vi "AxisSaveConfToFile.vi"(6 "Comunication":T1={"DeviceIDCtrl"=1, "ProtocolCtrl"=enum."Modbus RTU", "COMportCtrl"="", "IPCtrl"=""}, 7 "conf file path":path caption="selected path", 8 "error in (no error)":errorcluster, 9 "AditionalConfigOut":T2 {"UnitsControl" items=["mm", "°"]}, 10 "AxisWriteValuesIn":T3={"AxisTarget"=0.0, "AxisTargetVel"=1.0, "AxisStartReq"=FALSE, "AxisStopReq"=FALSE, "AxisClearReq"=FALSE, "AxisMovetype"=FALSE, "AxisMotorON"=FALSE, "MoveModeControl"=4, "AxisHomingVel"=1.0, "AxisAccDecc"=30.0} {"MoveModeControl" items=["Absolute", "Relative", "Velocity", "Homing"]}, 11 "AxisConfigurationIn":T4={"AxisHomeType"=1, "AxisBacklash"=0.0, "AxisGain"=1.0, "AxisOffset"=0.0, "AxisUnit"=1, "ReqConfRead"=FALSE, "ReqConfWrite"=FALSE, "AxisName"="", "AxisAccDecc"=0.0, "AxisHomeVel"=0.0} {"AxisUnit" items=["mm", "°"]; "AxisHomeType" items=["no homing"=0, "forward limit switch"=1, "backward limit switch"=2, "forward reference"=4, "backward reference"=8]}) -> (0 "error out":errorcluster)   [LabVIEW 2020, in "SMCD14_lib.lvlib"]
uses:
  SMCD14_lib.lvlib
  AxisConfiguration_typedef.ctl
  AxisWriteValues_typedef.ctl
  <vilib>/Utility/config.llb/Write Key (String).vi
  <vilib>/Utility/config.llb/Write Key (U32).vi
  <vilib>/Utility/config.llb/Write Key (Double).vi
  <vilib>/Utility/config.llb/Write Key (I32).vi
  <vilib>/Utility/config.llb/NI_LVConfig.lvlib
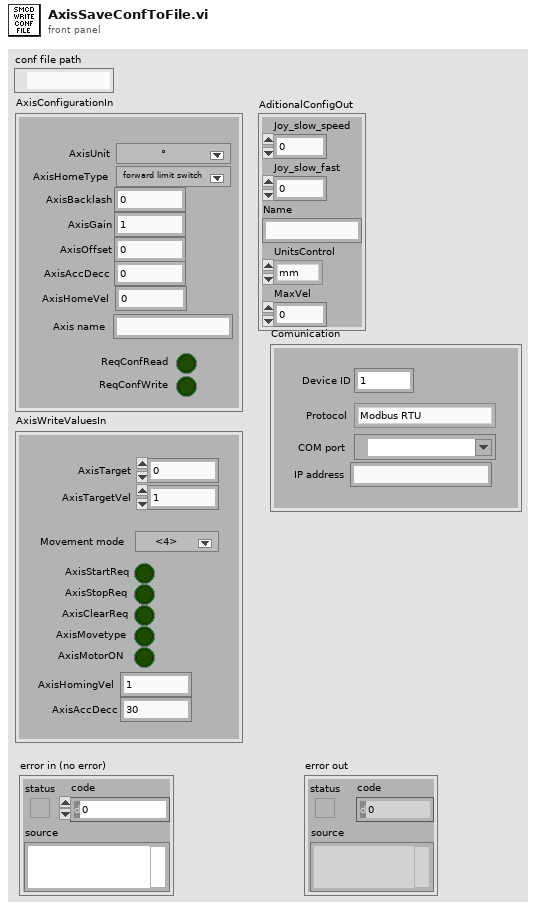
[diagram p1: front panel]
types:
  T1 = cluster{"DeviceIDCtrl":u16, "ProtocolCtrl":enum16{"Modbus RTU", "Modbus TCP", ""}, "COMportCtrl":refnum<visa-resource-name>, "IPCtrl":string}
  T2 = cluster{"Joy_slow_speed":sgl, "Joy_slow_fast":sgl, "Name":string, "UnitsControl":u16, "MaxVel":sgl}
  T3 = typedef "SMCD14_lib.lvlib/AxisWriteValues_typedef.ctl" = cluster{"AxisTarget":dbl, "AxisTargetVel":dbl, "AxisStartReq":bool, "AxisStopReq":bool, "AxisClearReq":bool, "AxisMovetype":bool, "AxisMotorON":bool, "MoveModeControl":u16, "AxisHomingVel":dbl, "AxisAccDecc":dbl}
  T4 = typedef "SMCD14_lib.lvlib/AxisConfiguration_typedef.ctl" = cluster{"AxisHomeType":u16, "AxisBacklash":dbl, "AxisGain":dbl, "AxisOffset":dbl, "AxisUnit":u16, "ReqConfRead":bool, "ReqConfWrite":bool, "AxisName":string, "AxisAccDecc":dbl, "AxisHomeVel":dbl}
  T5 = typedef "NI_LVConfig.lvlib/Config Data RefNum.ctl" = refnum<k1>
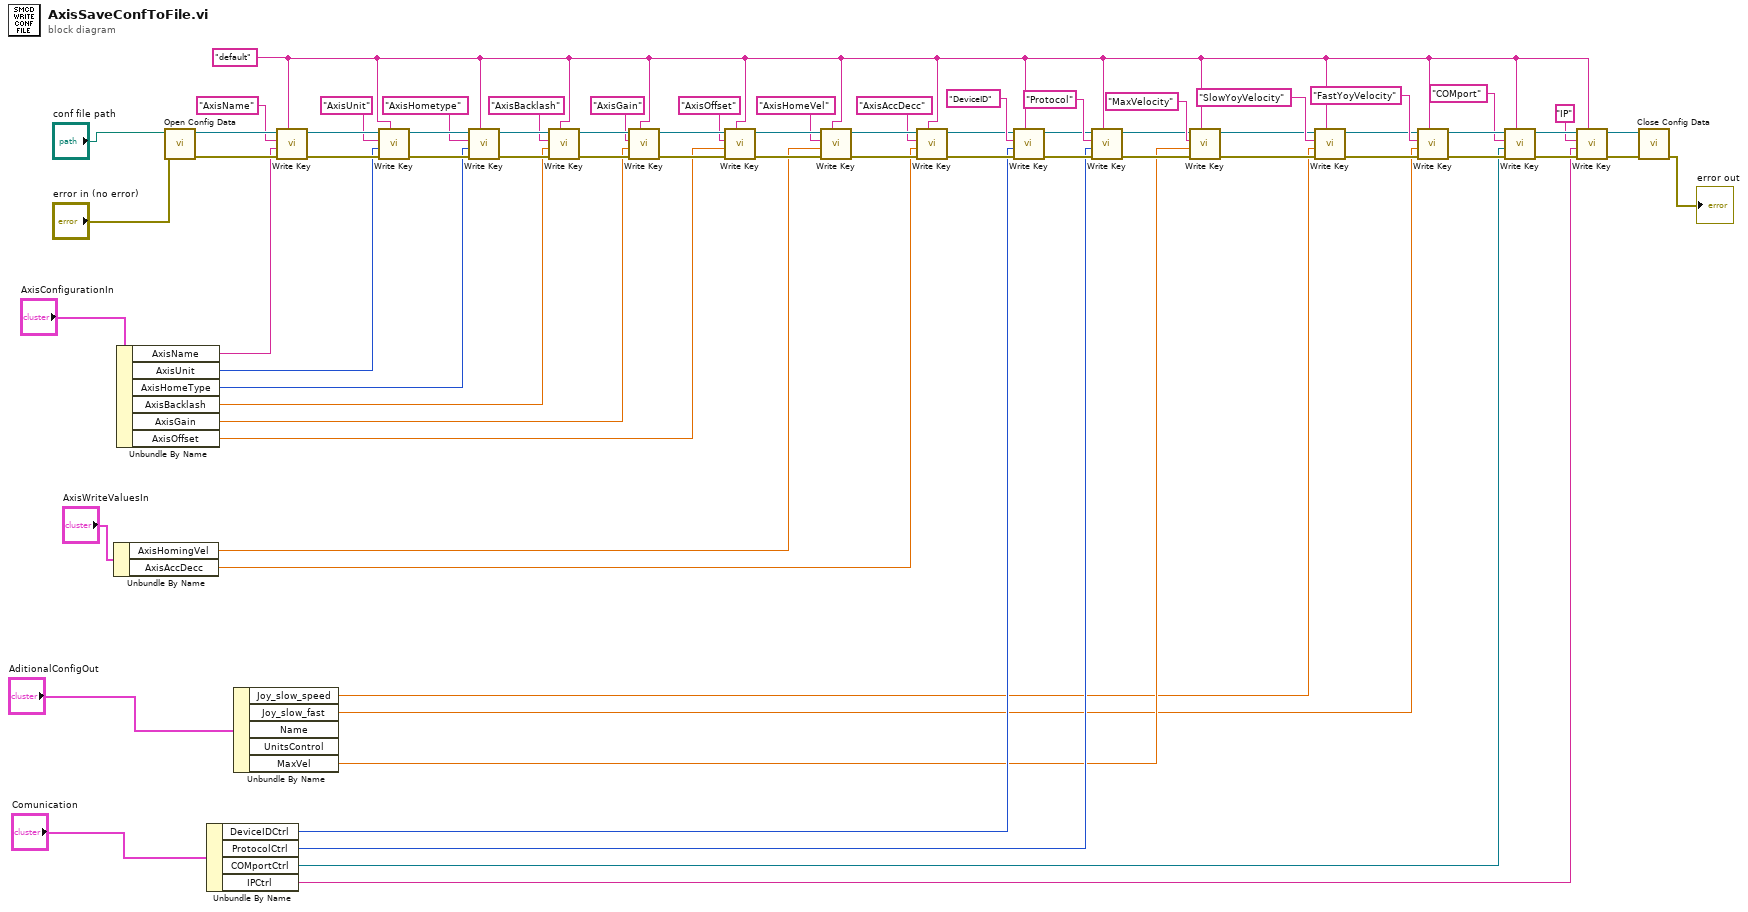
[diagram p0: block diagram]
diagram:
  w1 = "default" ("section")
  n1 = Unbundle By Name("AxisWriteValuesIn") -> ("AxisHomingVel"=w36:dbl, "AxisAccDecc"=w35:dbl)
  n2 = Unbundle By Name("AxisConfigurationIn") -> ("AxisName"=w43:string, "AxisUnit"=w42:u16, "AxisHomeType"=w41:u16, "AxisBacklash"=w40:dbl, "AxisGain"=w39:dbl, "AxisOffset"=w38:dbl)
  n3 = call <vilib>:"Open Config Data.vi"("error in (no error)"="error in (no error)", "configuration file path"="conf file path") -> ("error out"=w69:errorcluster, "refnum"=w70:T5)  [unwired: 7 in, 1 out]
  n4 = Unbundle By Name("Comunication") -> ("DeviceIDCtrl"=w14:u16, "ProtocolCtrl"=w13:enum16{"Modbus RTU", "Modbus TCP", ""}, "COMportCtrl"=w8:refnum<visa-resource-name>, "IPCtrl"=w2:string)
  n5 = Unbundle By Name("AditionalConfigOut") -> ("Joy_slow_speed"=w11:sgl, "Joy_slow_fast"=w10:sgl, "MaxVel"=w12:sgl)  [unwired: 2 out]
  n6 = call-poly <vilib>:"Write Key.vi"("section"=w1, "error in (no error)"=w69, "value"=w43, "key"="AxisName", "refnum"=w70) -> ("error out"=w61:errorcluster, "refnum out"=w67:T5)  [unwired: 4 in, 1 out]
  n7 = call-poly <vilib>:"Write Key.vi"("section"=w1, "error in (no error)"=w61, "value"=w42, "key"="AxisUnit", "refnum"=w67) -> ("error out"=w60:errorcluster, "refnum out"=w65:T5)  [unwired: 4 in, 1 out]
  n8 = call-poly <vilib>:"Write Key.vi"("section"=w1, "error in (no error)"=w60, "value"=w41, "key"="AxisHometype", "refnum"=w65) -> ("error out"=w59:errorcluster, "refnum out"=w63:T5)  [unwired: 4 in, 1 out]
  n9 = call-poly <vilib>:"Write Key.vi"("section"=w1, "error in (no error)"=w59, "value"=w40, "key"="AxisBacklash", "refnum"=w63) -> ("error out"=w57:errorcluster, "refnum out"=w58:T5)  [unwired: 4 in, 1 out]
  n10 = call-poly <vilib>:"Write Key.vi"("section"=w1, "error in (no error)"=w57, "value"=w39, "key"="AxisGain", "refnum"=w58) -> ("error out"=w54:errorcluster, "refnum out"=w55:T5)  [unwired: 4 in, 1 out]
  n11 = call-poly <vilib>:"Write Key.vi"("section"=w1, "error in (no error)"=w54, "value"=w38, "key"="AxisOffset", "refnum"=w55) -> ("error out"=w51:errorcluster, "refnum out"=w52:T5)  [unwired: 4 in, 1 out]
  n12 = call-poly <vilib>:"Write Key.vi"("section"=w1, "error in (no error)"=w51, "value"=w36, "key"="AxisHomeVel", "refnum"=w52) -> ("error out"=w47:errorcluster, "refnum out"=w48:T5)  [unwired: 4 in, 1 out]
  n13 = call-poly <vilib>:"Write Key.vi"("section"=w1, "error in (no error)"=w47, "value"=w35, "key"="AxisAccDecc", "refnum"=w48) -> ("error out"=w25:errorcluster, "refnum out"=w26:T5)  [unwired: 4 in, 1 out]
  n14 = call-poly <vilib>:"Write Key.vi"("section"=w1, "error in (no error)"=w25, "value"=w14, "key"="DeviceID", "refnum"=w26) -> ("error out"=w23:errorcluster, "refnum out"=w24:T5)  [unwired: 4 in, 1 out]
  n15 = call-poly <vilib>:"Write Key.vi"("section"=w1, "error in (no error)"=w23, "value"=w13, "key"="Protocol", "refnum"=w24) -> ("error out"=w21:errorcluster, "refnum out"=w22:T5)  [unwired: 4 in, 1 out]
  n16 = call-poly <vilib>:"Write Key.vi"("section"=w1, "error in (no error)"=w21, "value"=w12, "key"="MaxVelocity", "refnum"=w22) -> ("error out"=w18:errorcluster, "refnum out"=w20:T5)  [unwired: 4 in, 1 out]
  n17 = call-poly <vilib>:"Write Key.vi"("section"=w1, "error in (no error)"=w18, "value"=w11, "key"="SlowYoyVelocity", "refnum"=w20) -> ("error out"=w17:errorcluster, "refnum out"=w19:T5)  [unwired: 4 in, 1 out]
  n18 = call-poly <vilib>:"Write Key.vi"("section"=w1, "error in (no error)"=w17, "value"=w10, "key"="FastYoyVelocity", "refnum"=w19) -> ("error out"=w9:errorcluster, "refnum out"=w16:T5)  [unwired: 4 in, 1 out]
  n19 = call-poly <vilib>:"Write Key.vi"("section"=w1, "error in (no error)"=w9, "value"=w8, "key"="COMport", "refnum"=w16) -> ("error out"=w6:errorcluster, "refnum out"=w7:T5)  [unwired: 4 in, 1 out]
  n20 = call-poly <vilib>:"Write Key.vi"("section"=w1, "error in (no error)"=w6, "value"=w2, "key"="IP", "refnum"=w7) -> ("error out"=w4:errorcluster, "refnum out"=w5:T5)  [unwired: 4 in, 1 out]
  n21 = call <vilib>:"Close Config Data.vi"("error in (no error)"=w4, "refnum"=w5) -> ("error out"=→"error out":errorcluster)  [unwired: 8 in, 1 out]
